vi "fpga_send_data.vi"(7 "DMA":bool, 11 "data":T1) -> ()   [LabVIEW 2021]
doc: "When DMA is true, send data to the host computer."
uses:
  fpga_dtype_data.ctl
  fpga_dtype_sgl_8ch.ctl
  fpga_dtype_sgl_fb.ctl
  fpga_dtype_status.ctl
  fpga_dtype_index.ctl
  <vilib>/rvi/interface/RandomDataEmulation/nirviRandomDataMultiElementFPGAFIFO.vi
  <instcachedir>/0/nirviRandomDataMultiElementFPGAFIFO_3E9965BA1FAD4E7B8DABA31768A09B1F.lvgen/nirviRandomDataMultiElementFPGAFIFO_3E9965BA1FAD4E7B8DABA31768A09B1F_001.vi
  <vilib>/rvi/interface/RandomDataEmulation/niFpgaRandomDataHandleErrors.vi
  <vilib>/rvi/DataTransferAndStorage/Container/Common/niFpgaContainerExecOnDevCompGetState.vi
  <vilib>/rvi/Emulation/niFpgaSctlEmulationGetInTimedLoop.vi
  <vilib>/rvi/errors/niFpgaSetErrorForExecOnDevCompSimple.vi
  <vilib>/rvi/eio/common/nirviEmuReportErrorAndStop.vi
  <vilib>/rvi/interface/RandomDataEmulation/nirviRandomDataAcquireLock.vi
  <vilib>/rvi/interface/RandomDataEmulation/nirviRandomDataQueueStore.vi
  <vilib>/rvi/interface/RandomDataEmulation/nirviRandomDataReleaseLock.vi
  <vilib>/rvi/interface/RandomDataEmulation/nirviFPGAContextMergeError.vi
  <vilib>/rvi/interface/RandomDataEmulation/nirviRandomDataCheckExitLoopConditions.vi
  <vilib>/express/rvi/timingcommon/nirviCommon.vi
  <instcachedir>/0/nirviRandomDataMultiElementFPGAFIFO_3E9965BA1FAD4E7B8DABA31768A09B1F.lvgen/nirviRandomDataMultiElementFPGAFIFO_3E9965BA1FAD4E7B8DABA31768A09B1F_000.vi
  <vilib>/rvi/DataTransferAndStorage/Container/XNode/niFpgaContainer.xnode
  <vilib>/rvi/interface/RandomDataEmulation/nirviRandomDataFpgaMultiElementTemplate.vi
  <vilib>/rvi/FIFO/Fifo_Resource/niFpgaFifoEmulationRefInMultiElement.vi
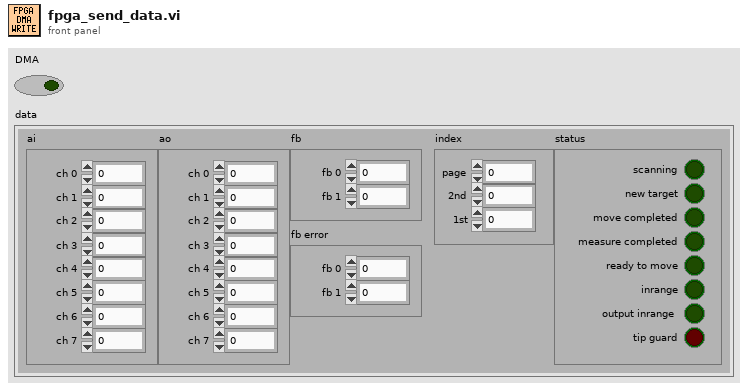
[diagram p1: front panel]
types:
  T1 = typedef "fpga_dtype_data.ctl" = cluster{"ai":T2, "ao":T2, "fb":T3, "fb error":T3, "status":T4, "index":T5}
  T2 = typedef "fpga_dtype_sgl_8ch.ctl" = cluster{"ch 0":sgl, "ch 1":sgl, "ch 2":sgl, "ch 3":sgl, "ch 4":sgl, "ch 5":sgl, "ch 6":sgl, "ch 7":sgl}
  T3 = typedef "fpga_dtype_sgl_fb.ctl" = cluster{"fb 0":sgl, "fb 1":sgl}
  T4 = typedef "fpga_dtype_status.ctl" = cluster{"scanning":bool, "new target":bool, "move completed":bool, "measure completed":bool, "inrange":bool, "ready to move":bool, "output inrange":bool, "tip guard":bool}
  T5 = typedef "fpga_dtype_index.ctl" = cluster{"page":i16, "2nd":i16, "1st":i16}
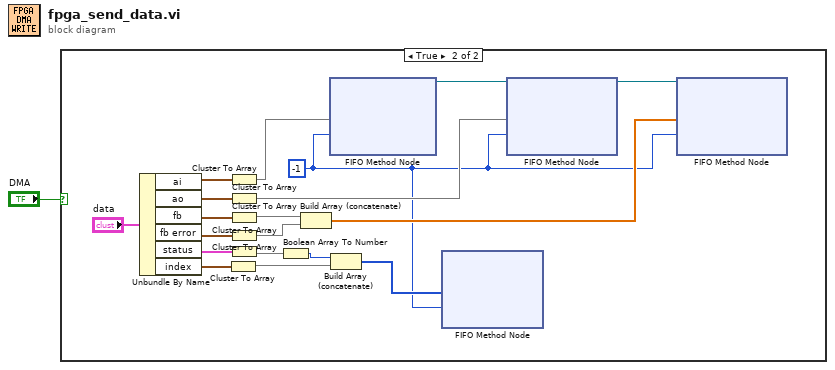
[diagram p0: block diagram]
diagram:
  n1 = case shown="True" "DMA" {
    frame False {
    }
    frame True {
      w2 = -1 ("Timeout")
      n2 = Unbundle By Name("data") -> ("ai"=w19:T2, "ao"=w18:T2, "fb"=w13:T3, "fb error"=w14:T3, "status"=w8:T4, "index"=w6:T5)
      n3 = Cluster To Array(cluster=w6) -> (array=w4:i16[])
      n4 = Cluster To Array(cluster=w19) -> (array=w17:sgl[])
      n5 = Cluster To Array(cluster=w18) -> (array=w16:sgl[])
      n6 = Cluster To Array(cluster=w13) -> (array=w12:sgl[])
      n7 = Cluster To Array(cluster=w14) -> (array=w11:sgl[])
      n8 = Cluster To Array(cluster=w8) -> (array=w7:bool[])
      n9 = Boolean Array To Number(Boolean array=w7) -> (number=w5:i16)
      n10 = Build Array (concatenate)(w12, w11) -> (w10:sgl[])
      n11 = xnode ("FIFO Method Node")("Element"=w17, "Timeout"=w2) -> ("FIFO Out"=w15:refnum<k21>)  [unwired: 1 in, 1 out]
      n12 = Build Array (concatenate)(w5, w4) -> (w3:i16[])
      n13 = xnode ("FIFO Method Node")("Element"=w3, "Timeout"=w2) -> ()  [unwired: 1 in, 2 out]
      n14 = xnode ("FIFO Method Node")("Element"=w16, "Timeout"=w2, "FIFO In"=w15) -> ("FIFO Out"=w9:refnum<k21>)  [unwired: 1 out]
      n15 = xnode ("FIFO Method Node")("Element"=w10, "Timeout"=w2, "FIFO In"=w9) -> ()  [unwired: 2 out]
    }
  }
